vi "Open.vi"(7 "Allow multiple opens?":bool, 8 "error in (no error)":errorcluster, 10 "Channel Names":tag[](array[tag])) -> (0 "error out":errorcluster, 3 "AO Ref Out":T1)   [LabVIEW 2021, in "AO.lvlib"]
doc: "Opens a reference to one or more analog output channels. You must open a reference before you write values to an analog output channel."
uses:
  <vilib>/myRIO/Instrument Drivers/Onboard IO/AO/AO.lvlib
  <vilib>/myRIO/Instrument Drivers/Onboard IO/AO/typedefs/AO Reference.ctl
  <vilib>/myRIO/Common/Instrument Driver Framework/Utilities/typedefs/myRIO Generic Hardware Reference.ctl
  <vilib>/myRIO/Common/Instrument Driver Framework/Utilities/typedefs/Hardware Version Enum.ctl
  <vilib>/myRIO/Common/Instrument Driver Framework/Utilities/typedefs/myRIO v1.0 Reference.ctl
  <vilib>/myRIO/Common/Instrument Driver Framework/Utilities/typedefs/Generic FPGA Reference.ctl
  <vilib>/myRIO/Common/Instrument Driver Framework/myRIO v1.0/AO/typedefs/AO Channels List.ctl
  <vilib>/myRIO/Common/Instrument Driver Framework/myRIO v1.0/AO/typedefs/AO Channels Enum.ctl
  <vilib>/myRIO/Common/Instrument Driver Framework/Utilities/typedefs/Analog Scaling Constants List.ctl
  <vilib>/myRIO/Common/Instrument Driver Framework/Utilities/typedefs/Analog Scaling Constants.ctl
  <vilib>/myRIO/Common/Instrument Driver Framework/Utilities/vis/Validate Channels.vi
  <vilib>/myRIO/Common/Instrument Driver Framework/myRIO v1.0/AO/vis/myRIO v1.0 Reserve AO.vi
  <vilib>/myRIO/Common/Instrument Driver Framework/roboRIO v1.0/AO/vis/roboRIO v1.0 Reserve AO.vi
  <vilib>/myRIO/Common/Instrument Driver Framework/ELVIS III v1.0/AO/vis/ELVIS III v1.0 Reserve AO.vi
  <vilib>/myRIO/Common/Instrument Driver Framework/myRIO v1.0/AO/vis/myRIO v1.0 Build MUX Configuration AO.vi
  <vilib>/myRIO/Common/Instrument Driver Framework/myRIO v1.0/Resource Manager/vis/myRIO v1.0 Reserve Channel List.vi
  <vilib>/myRIO/Common/Instrument Driver Framework/roboRIO v1.0/AO/vis/roboRIO v1.0 Build MUX Configuration AO.vi
  <vilib>/myRIO/Common/Instrument Driver Framework/roboRIO v1.0/Resource Manager/vis/roboRIO v1.0 Reserve Channel List.vi
  <vilib>/myRIO/Common/Instrument Driver Framework/ELVIS III v1.0/AO/vis/ELVIS III v1.0 Build MUX Configuration AO.vi
  <vilib>/myRIO/Common/Instrument Driver Framework/myRIO v1.0/Resource Manager/vis/myRIO v1.0 Reserve Channel.vi
  <vilib>/myRIO/Common/Instrument Driver Framework/myRIO v1.0/Resource Manager/vis/myRIO v1.0 Unreserve Channel.vi
  <vilib>/myRIO/Common/Instrument Driver Framework/roboRIO v1.0/Resource Manager/vis/roboRIO v1.0 Reserve Channel.vi
  <vilib>/myRIO/Common/Instrument Driver Framework/roboRIO v1.0/Resource Manager/vis/roboRIO v1.0 Unreserve Channel.vi
  <vilib>/myRIO/Common/Instrument Driver Framework/myRIO v1.0/Resource Manager/vis/myRIO v1.0 Build Mutex Name.vi
  <vilib>/myRIO/Common/Instrument Driver Framework/roboRIO v1.0/Resource Manager/vis/roboRIO v1.0 Build Mutex Name.vi
  <vilib>/Utility/VariantDataType/GetNumericInfo.vi
  <vilib>/myRIO/Common/Instrument Driver Framework/myRIO v1.0/AO/vis/myRIO v1.0 Get Scaling Constants AO.vi
  <vilib>/myRIO/Common/Instrument Driver Framework/Utilities/vis/IO Manager.vi
  <vilib>/myRIO/Common/Instrument Driver Framework/Utilities/vis/Configuration Manager.vi
  <vilib>/myRIO/Common/Instrument Driver Framework/myRIO v1.0/myRIO v1.0 Close.vi
  <vilib>/myRIO/Common/Instrument Driver Framework/roboRIO v1.0/AO/vis/roboRIO v1.0 Get Scaling Constants AO.vi
  <vilib>/myRIO/Common/Instrument Driver Framework/ELVIS III v1.0/Resource Manager/vis/ELVIS III v1.0 Reserve Channel List.vi
  <vilib>/userdefined/High Color/nirio_resource_hc.ctl
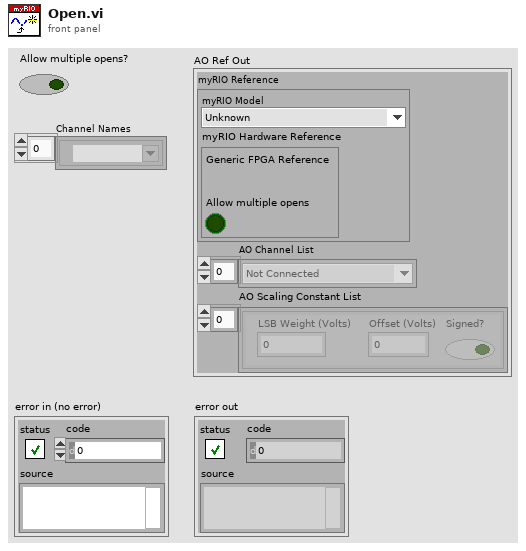
[diagram p1: front panel]
types:
  T1 = typedef "AO.lvlib/AO Reference.ctl" = cluster{"myRIO Reference":T2, "AO Channel List":T6, "AO Scaling Constant List":T8}
  T2 = typedef "myRIO Generic Hardware Reference.ctl" = cluster{"myRIO Model":T3, "myRIO Hardware Reference":T4}
  T3 = typedef "Hardware Version Enum.ctl" = enum16{"Unknown", "myRIO-1900", "myRIO-1950", "roboRIO", "NI ELVIS RIO CM", "ELVIS III"}
  T4 = typedef "myRIO v1.0 Reference.ctl" = cluster{"Generic FPGA Reference":T5, "Allow multiple opens":bool}
  T5 = typedef "Generic FPGA Reference.ctl" = refnum<k20>
  T6 = typedef "AO Channels List.ctl" = T7[]
  T7 = typedef "AO Channels Enum.ctl" = enum16{"Not Connected", "AudioOut/Left", "AudioOut/Right", "C/AO0", "C/AO1", "A/AO0", "A/AO1", "B/AO0", "B/AO1"}
  T8 = typedef "Analog Scaling Constants List.ctl" = T9[]
  T9 = typedef "Analog Scaling Constants.ctl" = cluster{"LSB Weight (Volts)":dbl, "Offset (Volts)":dbl, "Signed?":bool}
  T10 = typedef "nirio_resource_hc.ctl" = tag
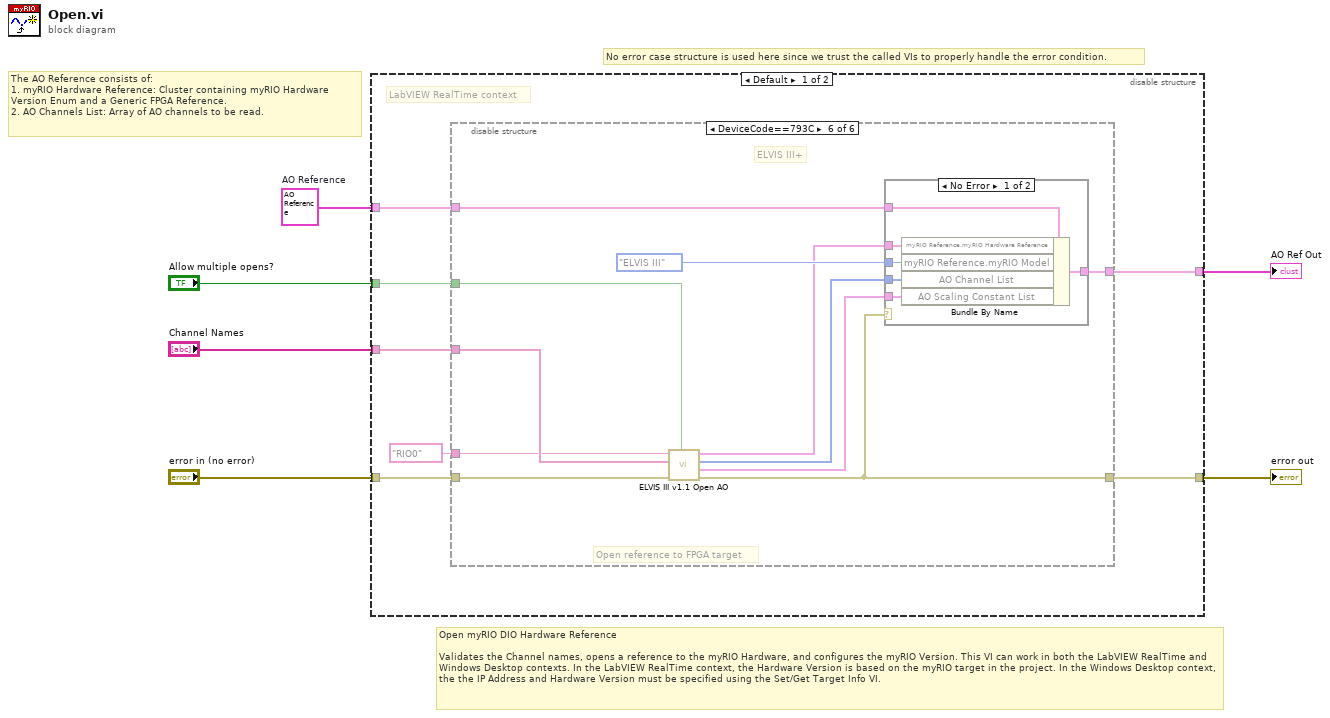
[diagram p0: block diagram]
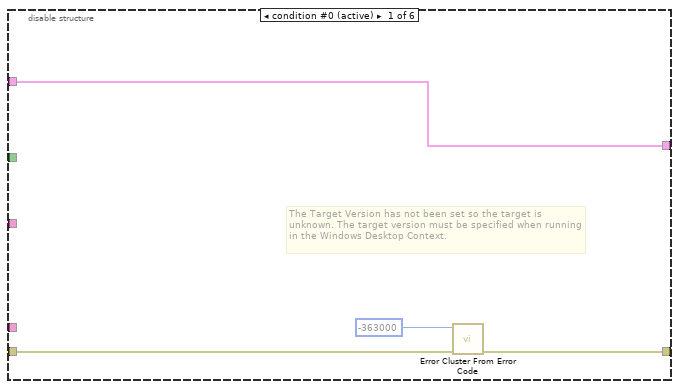
[diagram p2: hidden frame]
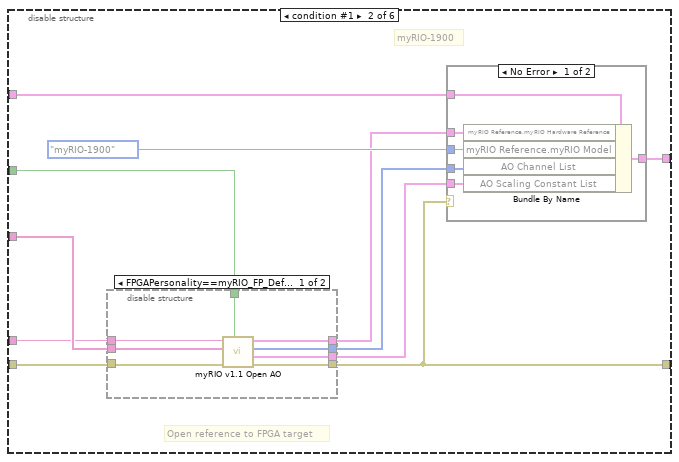
[diagram p3: hidden frame]
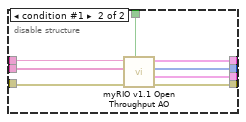
[diagram p4: hidden frame]
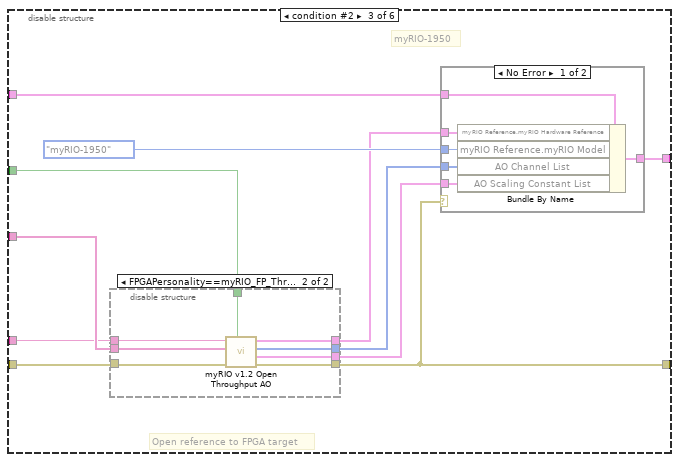
[diagram p6: hidden frame]
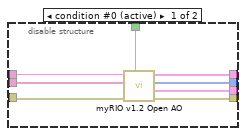
[diagram p7: hidden frame]
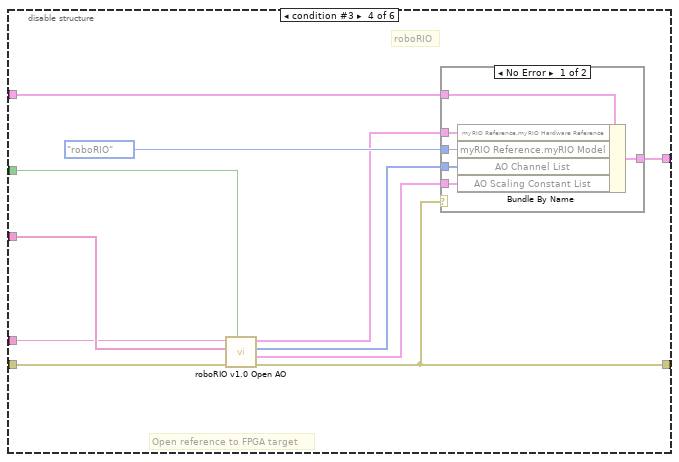
[diagram p9: hidden frame]
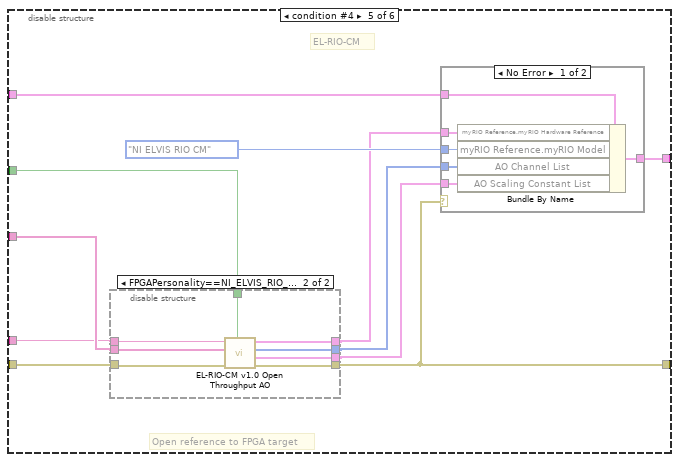
[diagram p11: hidden frame]
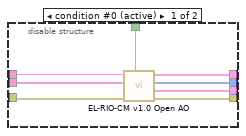
[diagram p12: hidden frame]
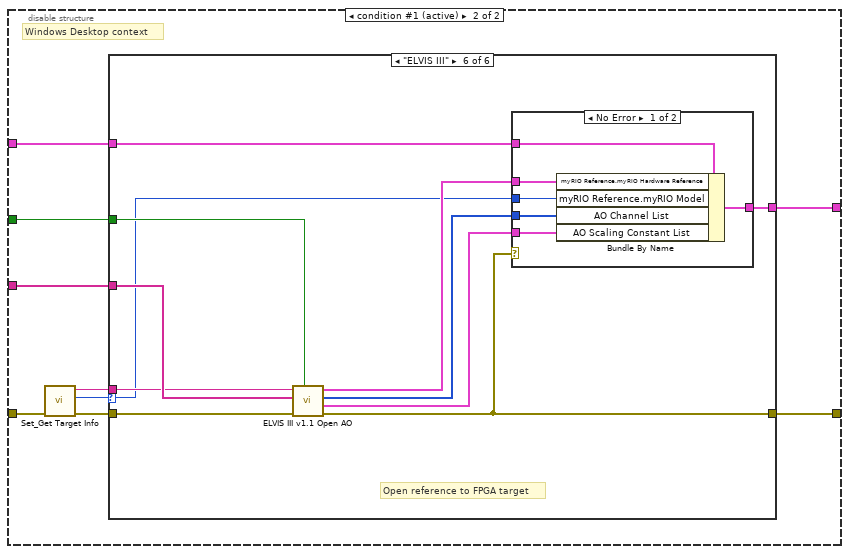
[diagram p15: hidden frame]
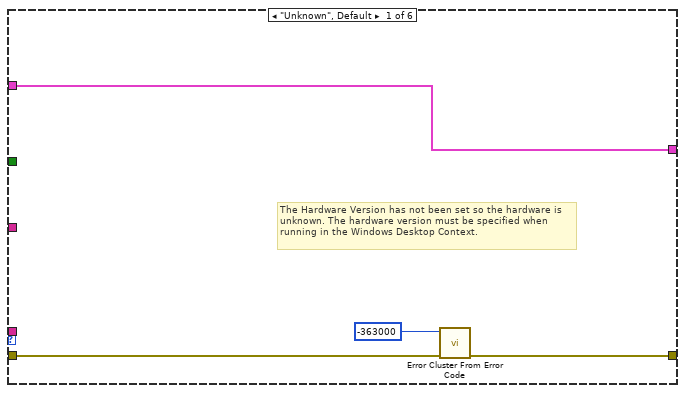
[diagram p16: hidden frame]
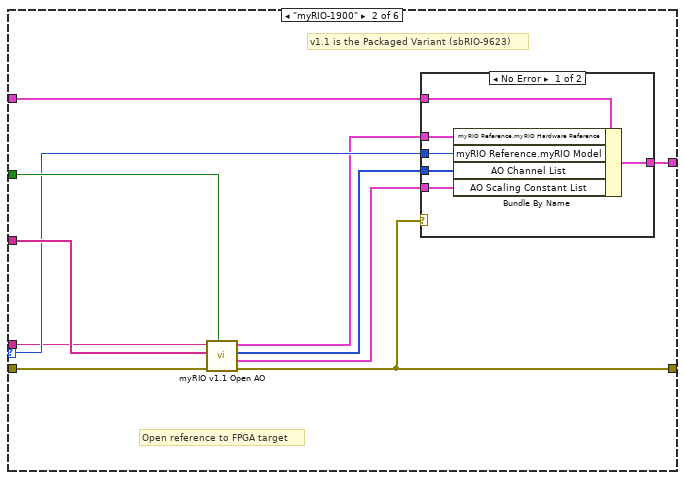
[diagram p17: hidden frame]
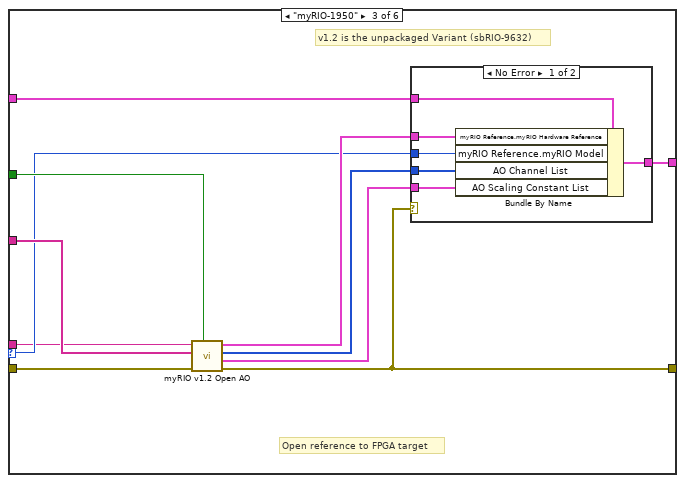
[diagram p19: hidden frame]
diagram:
  w6 = T1 {"myRIO Reference"={"myRIO Model"=enum."Unknown", "myRIO Hardware Reference"={"Generic FPGA Reference"=refnum, "Allow multiple opens"=FALSE}}, "AO Channel List"=[], "AO Scaling Constant List"=[]}  # AO Reference
  # "No error case structure is used here since we trust the called VIs to properly handle the error condition."
  # "Open myRIO DIO Hardware Reference\n\nValidates the Channel names, opens a reference to the myRIO Hardware, and configures the myRIO Version. This VI can work in both the LabVIEW RealTime and Windows Desktop contexts. In the LabVIEW RealTime context, the Hardware Version is based on the myRIO target in the project. In the Windows Desktop context, the the IP Address and Hardware Version must be specified using the Set/Get Target Info VI."
  # "The AO Reference consists of:\n1. myRIO Hardware Reference: Cluster containing myRIO Hardware Version Enum and a Generic FPGA Reference.\n2. AO Channels List: Array of AO channels to be read."
  n1 = disable-structure shown="Default" {
    disable-tunnel: [w13 w163] -> w2
    disable-tunnel: "Channel Names" -> [w12 w160]
    disable-tunnel: "Allow multiple opens?" -> [w11 w162]
    disable-tunnel: [w10 w161] -> w1
    disable-tunnel: "error in (no error)" -> [w9 w159]
    disable-tunnel: w6 -> [w8 w158]
    frame condition #0 {
      # "LabVIEW RealTime context"
      n2 = disable-structure shown="DeviceCode==793C" {
        disable-tunnel: [w17 w20 w54 w88 w111 w139] -> w13
        disable-tunnel: w12 -> [_ w28 w62 w96 w106 w142]
        disable-tunnel: w11 -> [_ w24 w61 w95 w104 w143]
        disable-tunnel: [w14 w27 w60 w94 w114 w138] -> w10
        disable-tunnel: w9 -> [w16 w25 w58 w92 w107 w140]
        disable-tunnel: w8 -> [w14 w23 w57 w91 w112 w144]
        disable-tunnel: T10 "RIO0" ("Resource name") -> [_ w21 w55 w89 w105 w141]
        frame condition #0 (active) {
          # "The Target Version has not been set so the target is unknown. The target version must be specified when running in the Windows Desktop Context."
          n3 = call <vilib>:"Error Cluster From Error Code.vi"("error in (no error)"=w16, "error code (0)"=-363000) -> ("error out"=w17:errorcluster)  [unwired: 7 in]
        }
        frame condition #1 {
          # "myRIO-1900"
          # "Open reference to FPGA target"
          n4 = disable-structure shown="FPGAPersonality==myRIO_FP_Default, Default" {
            disable-tunnel: w28 -> [w36 w44]
            disable-tunnel: w25 -> [w35 w43]
            disable-tunnel: w24 -> [w34 w42]
            disable-tunnel: [w33 w41] -> w22
            disable-tunnel: w21 -> [w32 w40]
            disable-tunnel: [w31 w39] -> w20
            disable-tunnel: [w30 w38] -> w19
            disable-tunnel: [w29 w37] -> w18
            frame condition #0 (active) {
              n5 = call <vilib>:"myRIO v1.1 Open AO.vi"("Allow multiple opens?"=w34, "error in (no error)"=w35, "Channel Names"=w36, "Resource name"=w32) -> ("error out"=w31:errorcluster, "AO Scale Constants List"=w29:T8, "AO Channel List"=w33:T6, "myRIO Ref Out"=w30:T4)  [unwired: 4 in]
            }
            frame condition #1 {
              n6 = call <vilib>:"myRIO v1.1 Open Throughput AO.vi"("Allow multiple opens?"=w42, "error in (no error)"=w43, "Channel Names"=w44, "Resource name"=w40) -> ("error out"=w39:errorcluster, "AO Scale Constants List"=w37:T8, "AO Channel List"=w41:T6, "myRIO Ref Out"=w38:T4)  [unwired: 4 in]
            }
          }
          n7 = case shown="No Error" w20 {
            tunnel: [w50 w51] -> w27
            tunnel: Hardware_Version_Enum."myRIO-1900" ("Hardware Version Enum") -> [w49 _]
            tunnel: w23 -> [w48 w51]
            tunnel: w22 -> [w47 _]
            tunnel: w19 -> [w46 _]
            tunnel: w18 -> [w45 _]
            frame No Error {
              n8 = Bundle By Name(cluster=w48, "myRIO Reference.myRIO Hardware Reference"=w46, "myRIO Reference.myRIO Model"=w49, "AO Channel List"=w47, "AO Scaling Constant List"=w45) -> (w50:T1)
            }
            frame Error {
            }
          }
        }
        frame condition #2 {
          # "myRIO-1950"
          # "Open reference to FPGA target"
          n9 = disable-structure shown="FPGAPersonality==myRIO_FP_Throughput" {
            disable-tunnel: w62 -> [w70 w78]
            disable-tunnel: w61 -> [w69 w77]
            disable-tunnel: w58 -> [w68 w76]
            disable-tunnel: [w67 w75] -> w56
            disable-tunnel: w55 -> [w66 w74]
            disable-tunnel: [w65 w73] -> w54
            disable-tunnel: [w64 w72] -> w53
            disable-tunnel: [w63 w71] -> w52
            frame condition #0 (active) {
              n10 = call <vilib>:"myRIO v1.2 Open AO.vi"("Allow multiple opens?"=w69, "error in (no error)"=w68, "Channel Names"=w70, "Resource name"=w66) -> ("error out"=w65:errorcluster, "AO Scale Constants List"=w63:T8, "AO Channel List"=w67:T6, "myRIO Ref Out"=w64:T4)  [unwired: 4 in]
            }
            frame condition #1 {
              n11 = call <vilib>:"myRIO v1.2 Open Throughput AO.vi"("Allow multiple opens?"=w77, "error in (no error)"=w76, "Channel Names"=w78, "Resource name"=w74) -> ("error out"=w73:errorcluster, "AO Scale Constants List"=w71:T8, "AO Channel List"=w75:T6, "myRIO Ref Out"=w72:T4)  [unwired: 4 in]
            }
          }
          n12 = case shown="No Error" w54 {
            tunnel: [w84 w85] -> w60
            tunnel: Hardware_Version_Enum."myRIO-1950" ("Hardware Version Enum") -> [w83 _]
            tunnel: w57 -> [w82 w85]
            tunnel: w56 -> [w81 _]
            tunnel: w53 -> [w80 _]
            tunnel: w52 -> [w79 _]
            frame No Error {
              n13 = Bundle By Name(cluster=w82, "myRIO Reference.myRIO Hardware Reference"=w80, "myRIO Reference.myRIO Model"=w83, "AO Channel List"=w81, "AO Scaling Constant List"=w79) -> (w84:T1)
            }
            frame Error {
            }
          }
        }
        frame condition #3 {
          # "roboRIO"
          # "Open reference to FPGA target"
          n14 = call <vilib>:"roboRIO v1.0 Open AO.vi"("Allow multiple opens?"=w95, "error in (no error)"=w92, "Channel Names"=w96, "Resource name"=w89) -> ("error out"=w88:errorcluster, "AO Scale Constants List"=w86:T8, "AO Channel List"=w90:T6, "myRIO Ref Out"=w87:T4)  [unwired: 4 in]
          n15 = case shown="No Error" w88 {
            tunnel: [w102 w103] -> w94
            tunnel: Hardware_Version_Enum."roboRIO" ("Hardware Version Enum") -> [w101 _]
            tunnel: w91 -> [w100 w103]
            tunnel: w90 -> [w99 _]
            tunnel: w87 -> [w98 _]
            tunnel: w86 -> [w97 _]
            frame No Error {
              n16 = Bundle By Name(cluster=w100, "myRIO Reference.myRIO Hardware Reference"=w98, "myRIO Reference.myRIO Model"=w101, "AO Channel List"=w99, "AO Scaling Constant List"=w97) -> (w102:T1)
            }
            frame Error {
            }
          }
        }
        frame condition #4 {
          # "EL-RIO-CM"
          # "Open reference to FPGA target"
          n17 = disable-structure shown="FPGAPersonality==NI_ELVIS_RIO_CM_FP_Throughput" {
            disable-tunnel: w106 -> [w122 w125]
            disable-tunnel: w104 -> [w121 w123]
            disable-tunnel: w107 -> [w120 w124]
            disable-tunnel: [w119 w128] -> w109
            disable-tunnel: w105 -> [w118 w126]
            disable-tunnel: [w117 w130] -> w111
            disable-tunnel: [w116 w127] -> w108
            disable-tunnel: [w115 w129] -> w110
            frame condition #0 (active) {
              n18 = call <vilib>:"EL-RIO-CM v1.0 Open AO.vi"("Allow multiple opens?"=w121, "error in (no error)"=w120, "Channel Names"=w122, "Resource name"=w118) -> ("error out"=w117:errorcluster, "AO Scale Constants List"=w115:T8, "AO Channel List"=w119:T6, "myRIO Ref Out"=w116:T4)  [unwired: 4 in]
            }
            frame condition #1 {
              n19 = call <vilib>:"EL-RIO-CM v1.0 Open Throughput AO.vi"("Allow multiple opens?"=w123, "error in (no error)"=w124, "Channel Names"=w125, "Resource name"=w126) -> ("error out"=w130:errorcluster, "AO Scale Constants List"=w129:T8, "AO Channel List"=w128:T6, "myRIO Ref Out"=w127:T4)  [unwired: 4 in]
            }
          }
          n20 = case shown="No Error" w111 {
            tunnel: [w136 w137] -> w114
            tunnel: Hardware_Version_Enum."NI ELVIS RIO CM" ("Hardware Version Enum") -> [w135 _]
            tunnel: w112 -> [w134 w137]
            tunnel: w109 -> [w133 _]
            tunnel: w108 -> [w132 _]
            tunnel: w110 -> [w131 _]
            frame No Error {
              n21 = Bundle By Name(cluster=w134, "myRIO Reference.myRIO Hardware Reference"=w132, "myRIO Reference.myRIO Model"=w135, "AO Channel List"=w133, "AO Scaling Constant List"=w131) -> (w136:T1)
            }
            frame Error {
            }
          }
        }
        frame condition #5 {
          # "ELVIS III+"
          # "Open reference to FPGA target"
          n22 = call <vilib>:"ELVIS III v1.1 Open AO.vi"("Allow multiple opens?"=w143, "error in (no error)"=w140, "Channel Names"=w142, "Resource name"=w141) -> ("error out"=w139:errorcluster, "AO Scale Constants List"=w147:T8, "AO Channel List"=w146:T6, "myRIO Ref Out"=w145:T4)  [unwired: 4 in]
          n23 = case shown="No Error" w139 {
            tunnel: [w154 w155] -> w138
            tunnel: Hardware_Version_Enum."ELVIS III" ("Hardware Version Enum") -> [w153 _]
            tunnel: w144 -> [w152 w155]
            tunnel: w146 -> [w151 _]
            tunnel: w145 -> [w150 _]
            tunnel: w147 -> [w149 _]
            frame No Error {
              n24 = Bundle By Name(cluster=w152, "myRIO Reference.myRIO Hardware Reference"=w150, "myRIO Reference.myRIO Model"=w153, "AO Channel List"=w151, "AO Scaling Constant List"=w149) -> (w154:T1)
            }
            frame Error {
            }
          }
        }
      }
    }
    frame condition #1 (active) {
      # "Windows Desktop context"
      n25 = call <vilib>:"Set_Get Target Info.vi"() -> ("Hardware Version"=w156:T3, "IP Address"=w157:string)  [unwired: 9 in, 1 out]
      n26 = case shown="\"ELVIS III\"" w156 {
        selector: w156 -> [_ w175 w193 w211 w229 w243]
        tunnel: [w167 w170 w187 w205 w223 w241] -> w163
        tunnel: w160 -> [_ w178 w196 w214 w232 w245]
        tunnel: w162 -> [_ w177 w195 w213 w231 w246]
        tunnel: [w164 w176 w188 w206 w224 w240] -> w161
        tunnel: w159 -> [w165 w171 w192 w210 w228 w242]
        tunnel: w157 -> [_ w174 w191 w209 w227 w244]
        tunnel: w158 -> [w164 w173 w190 w208 w226 w247]
        frame "Unknown", Default {
          # "The Hardware Version has not been set so the hardware is unknown. The hardware version must be specified when running in the Windows Desktop Context."
          n27 = call <vilib>:"Error Cluster From Error Code.vi"("error in (no error)"=w165, "error code (0)"=-363000) -> ("error out"=w167:errorcluster)  [unwired: 7 in]
        }
        frame "myRIO-1900" {
          # "v1.1 is the Packaged Variant (sbRIO-9623)"
          # "Open reference to FPGA target"
          n28 = call <vilib>:"myRIO v1.1 Open AO.vi"("Allow multiple opens?"=w177, "error in (no error)"=w171, "Channel Names"=w178, "Resource name"=w174) -> ("error out"=w170:errorcluster, "AO Scale Constants List"=w168:T8, "AO Channel List"=w172:T6, "myRIO Ref Out"=w169:T4)  [unwired: 4 in]
          n29 = case shown="No Error" w170 {
            tunnel: [w184 w185] -> w176
            tunnel: w175 -> [w183 _]
            tunnel: w173 -> [w182 w185]
            tunnel: w172 -> [w181 _]
            tunnel: w169 -> [w180 _]
            tunnel: w168 -> [w179 _]
            frame No Error {
              n30 = Bundle By Name(cluster=w182, "myRIO Reference.myRIO Hardware Reference"=w180, "myRIO Reference.myRIO Model"=w183, "AO Channel List"=w181, "AO Scaling Constant List"=w179) -> (w184:T1)
            }
            frame Error {
            }
          }
        }
        frame "myRIO-1950" {
          # "v1.2 is the unpackaged Variant (sbRIO-9632)"
          # "Open reference to FPGA target"
          n31 = call <vilib>:"myRIO v1.2 Open AO.vi"("Allow multiple opens?"=w195, "error in (no error)"=w192, "Channel Names"=w196, "Resource name"=w191) -> ("error out"=w187:errorcluster, "AO Scale Constants List"=w186:T8, "AO Channel List"=w189:T6, "myRIO Ref Out"=w194:T4)  [unwired: 4 in]
          n32 = case shown="No Error" w187 {
            tunnel: w194 -> [w198 _]
            tunnel: w193 -> [w202 _]
            tunnel: w190 -> [w201 w203]
            tunnel: w189 -> [w200 _]
            tunnel: [w199 w203] -> w188
            tunnel: w186 -> [w197 _]
            frame No Error {
              n33 = Bundle By Name(cluster=w201, "myRIO Reference.myRIO Hardware Reference"=w198, "myRIO Reference.myRIO Model"=w202, "AO Channel List"=w200, "AO Scaling Constant List"=w197) -> (w199:T1)
            }
            frame Error {
            }
          }
        }
        frame "roboRIO" {
          # "Open reference to FPGA target"
          n34 = call <vilib>:"roboRIO v1.0 Open AO.vi"("Allow multiple opens?"=w213, "error in (no error)"=w210, "Channel Names"=w214, "Resource name"=w209) -> ("error out"=w205:errorcluster, "AO Scale Constants List"=w204:T8, "AO Channel List"=w207:T6, "myRIO Ref Out"=w212:T4)  [unwired: 4 in]
          n35 = case shown="No Error" w205 {
            tunnel: w212 -> [w216 _]
            tunnel: w211 -> [w220 _]
            tunnel: w208 -> [w219 w221]
            tunnel: w207 -> [w218 _]
            tunnel: [w217 w221] -> w206
            tunnel: w204 -> [w215 _]
            frame No Error {
              n36 = Bundle By Name(cluster=w219, "myRIO Reference.myRIO Hardware Reference"=w216, "myRIO Reference.myRIO Model"=w220, "AO Channel List"=w218, "AO Scaling Constant List"=w215) -> (w217:T1)
            }
            frame Error {
            }
          }
        }
        frame "NI ELVIS RIO CM" {
          # "Open reference to FPGA target"
          n37 = call <vilib>:"EL-RIO-CM v1.0 Open AO.vi"("Allow multiple opens?"=w231, "error in (no error)"=w228, "Channel Names"=w232, "Resource name"=w227) -> ("error out"=w223:errorcluster, "AO Scale Constants List"=w222:T8, "AO Channel List"=w225:T6, "myRIO Ref Out"=w230:T4)  [unwired: 4 in]
          n38 = case shown="No Error" w223 {
            tunnel: w230 -> [w234 _]
            tunnel: w229 -> [w238 _]
            tunnel: w226 -> [w237 w239]
            tunnel: w225 -> [w236 _]
            tunnel: [w235 w239] -> w224
            tunnel: w222 -> [w233 _]
            frame No Error {
              n39 = Bundle By Name(cluster=w237, "myRIO Reference.myRIO Hardware Reference"=w234, "myRIO Reference.myRIO Model"=w238, "AO Channel List"=w236, "AO Scaling Constant List"=w233) -> (w235:T1)
            }
            frame Error {
            }
          }
        }
        frame "ELVIS III" {
          # "Open reference to FPGA target"
          n40 = call <vilib>:"ELVIS III v1.1 Open AO.vi"("Allow multiple opens?"=w246, "error in (no error)"=w242, "Channel Names"=w245, "Resource name"=w244) -> ("error out"=w241:errorcluster, "AO Scale Constants List"=w248:T8, "AO Channel List"=w249:T6, "myRIO Ref Out"=w250:T4)  [unwired: 4 in]
          n41 = case shown="No Error" w241 {
            tunnel: w250 -> [w252 _]
            tunnel: w243 -> [w256 _]
            tunnel: w247 -> [w255 w257]
            tunnel: w249 -> [w254 _]
            tunnel: [w253 w257] -> w240
            tunnel: w248 -> [w251 _]
            frame No Error {
              n42 = Bundle By Name(cluster=w255, "myRIO Reference.myRIO Hardware Reference"=w252, "myRIO Reference.myRIO Model"=w256, "AO Channel List"=w254, "AO Scaling Constant List"=w251) -> (w253:T1)
            }
            frame Error {
            }
          }
        }
      }
    }
  }
  "AO Ref Out" <- w1
  "error out" <- w2
